vi "Pre Launch Init.vi"(11 "TableLogger_CSV_Actor in":refnum<class "TableLogger_CSV_Actor.lvclass">) -> (0 "error out":errorcluster, 3 "TableLogger_CSV_Actor out":refnum<class "TableLogger_CSV_Actor.lvclass">)   [LabVIEW 2014, in "TableLogger_CSV_Actor.lvlib" / "TableLogger_CSV_Actor.lvclass"]
doc: "(<B>Filename</B>: Actor Framework.lvlib:Actor.lvclass:Pre Launch Init.vi)\n\nDefines behavior that occurs after the Launch Nested Actor method is invoked but before the actor's Actor Core method begins running.\n\nBy default, this method does nothing. A descendant class may override it to define behavior."
uses:
  TableLogger_CSV_Actor.lvclass
  TableLogger_CSV_Actor.lvclass/TableLogger_CSV_Actor.ctl
  <userlib>/_OpenG.lib/file/file.llb/Strip Path - Traditional__ogtk.vi
  <userlib>/_OpenG.lib/file/file.llb/File Exists - Scalar__ogtk.vi
  <userlib>/_OpenG.lib/file/file.llb/Build Path - Traditional__ogtk.vi
  TableLogger_Actor/TableLogger_Actor/TableLogger_Actor.lvclass
panel:
  # "Connector Pane"
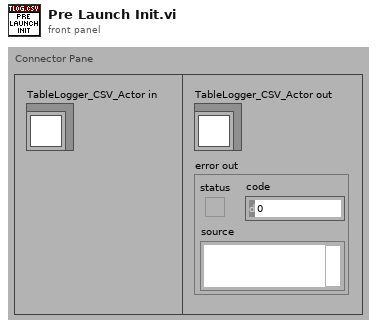
[diagram p1: front panel]
types:
  T1 = typedef "TableLogger_Actor.lvlib/TableLoggerConfig.ctl" = cluster{"TableLogger":T2, "DB File Path":path, "DB Backup Config":T3}
  T2 = typedef "TableLogger_Actor.lvlib/TableLoggerTypes.ctl" = enum16{"CSV Logger", "SQLite Logger"}
  T3 = typedef "TableLogger_Actor.lvlib/TableLoggerBackupConfig.ctl" = cluster{"Directory":path, "UTC Time Format":bool, "On Launch":bool, "Interval (Hours)":dbl, "Size Multiples (Bytes)":i32}
  T4 = typedef "Type Descriptor Enumeration__ogtk.ctl" = enum8{"<Null>", "I8", "I16", "I32", "I64", "U8", "U16", "U32", "U64", "SGL", "DBL", "EXT", "CSG", "CDB", "CXT", "0x0F", "0x10", "0x11", "0x12", "0x13", "0x14", "Enum U8", "Enum U16", "Enum U32", "Enum U64", "SGL PQ", "DBL PQ", "EXT PQ", "CSG PQ", "CDB PQ", "CXT PQ", "0x1F", "0x20", "Boolean", "0x22", "0x23", "0x24", "0x25", "0x26", "0x27", "0x28", "0x29", "0x2A", "0x2B", "0x2C", "0x2D", "0x2E", "0x2F", "String", "0x31", "Path", "Pict", "0x34", "0x35", "0x36", "DAQ", "0x38", "0x39", "0x3A", "0x3B", "0x3C", "0x3D", "0x3E", "0x3F", "Array", "0x41", "0x42", "0x43", "0x44", "0x45", "0x46", "0x47", "0x48", "0x49", "0x4A", "0x4B", "0x4C", "0x4D", "0x4E", "0x4F", "Cluster", "0x51", "0x52", "Variant", "Waveform", "0x55", "0x56", "0x57", "0x58", "0x59", "0x5A", "0x5B", "0x5C", "0x5D", "0x5E", "0x5F", "0x60", "0x61", "0x62", "0x63", "0x64", "0x65", "0x66", "0x67", "0x68", "0x69", "0x6A", "0x6B", "0x6C", "0x6D", "0x6E", "0x6F", "Refnum"}
  T5 = enum16{"open", "replace", "create", "open or create", "replace or create", "replace or create with confirmation"}
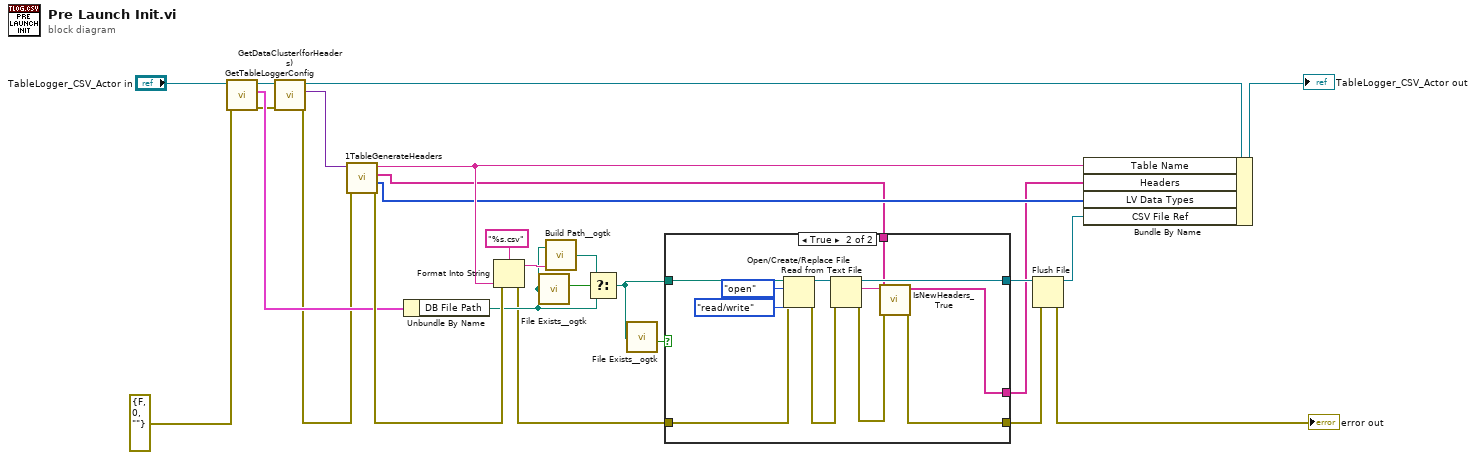
[diagram p0: block diagram]
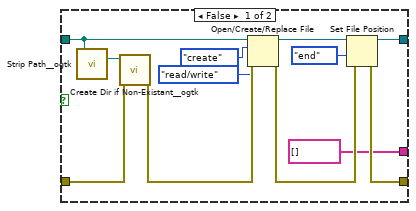
[diagram p2: hidden frame]
diagram:
  n1 = call-dynamic "GetTableLoggerConfig.vi"("error in (no error)"=errorcluster {"status"=FALSE, "code"=0, "source"=""}, "object in"="TableLogger_CSV_Actor in") -> ("error out"=w3:errorcluster, "TableLogger Config"=w5:T1, "object out"=w6:refnum<class "TableLogger_CSV_Actor.lvclass">)  [unwired: 7 in]
  n2 = call "GetDataCluster(forHeaders).vi"("error in (no error)"=w3, "object in"=w6) -> ("error out"=w1:errorcluster, "Data Cluster (for Headers)"=w4:variant, "object out"=w7:refnum<class "TableLogger_CSV_Actor.lvclass">)  [unwired: 7 in]
  n3 = call "1TableGenerateHeaders.vi"("error in (no error)"=w1, "Cluster Variant"=w4) -> ("error out"=w20:errorcluster, "LV Data Types"=w15:T4[], "Headers"=w12:string[], "Table Name"=w19:string)  [unwired: 6 in]
  n4 = Unbundle By Name(w5) -> ("DB File Path"=w18:path)
  n5 = Format Into String(format string="%s.csv", error in=w20, w19) -> (resulting string=w23:string, error out=w17:errorcluster)  [unwired: 1 in]
  n6 = call-poly <userlib>:"File Exists__ogtk.vi"("file path"=w18) -> ("is directory"=w24:bool)  [unwired: 6 in, 1 out]
  n7 = call-poly <userlib>:"Build Path__ogtk.vi"("name or relative path"=w23, "base path"=w18) -> ("appended path"=w21:path)
  n8 = Select(t=w21, s=w24, f=w18) -> (s? t:f=w14:path)
  n9 = call-poly <userlib>:"File Exists__ogtk.vi"("file path"=w14) -> ("exists"=w13:bool)  [unwired: 6 in, 1 out]
  n10 = case shown="True" w13 {
    tunnel: w17 -> [w36 w47]
    tunnel: [w28 w40] -> w11
    tunnel: [w30 w42] -> w10
    tunnel: w14 -> [w33 w50]
    tunnel: w12 -> [_ w41]
    tunnel: [string[] [] ("Headers") w39] -> w9
    frame False {
      n11 = call-poly <userlib>:"Strip Path__ogtk.vi"("path"=w33) -> ("stripped path"=w37:path)  [unwired: 1 out]
      n12 = call <userlib>:"Create Dir if Non-Existant__ogtk.vi"("error in (no error)"=w36, "Directory Path"=w37) -> ("error out"=w35:errorcluster)  [unwired: 7 in, 2 out]
      n13 = Open/Create/Replace File(file path (use dialog)=w33, error in=w35, operation (0:open)=T5."create", access (0:read/write)=enum16{"read/write", "read-only", "write-only"}."read/write") -> (refnum out=w31:refnum<file>, error out=w29:errorcluster)  [unwired: 2 in, 1 out]
      n14 = Set File Position(refnum=w31, from (0:start)=enum16{"start", "end", "current"}."end", error in=w29) -> (refnum out=w30:refnum<file>, error out=w28:errorcluster)  [unwired: 1 in]
    }
    frame True {
      n15 = Open/Create/Replace File(file path (use dialog)=w50, error in=w47, operation (0:open)=T5."open", access (0:read/write)=enum16{"read/write", "read-only", "write-only"}."read/write") -> (refnum out=w46:refnum<file>, error out=w43:errorcluster)  [unwired: 2 in, 1 out]
      n16 = Read from Text File(file (use dialog)=w46, error in=w43) -> (refnum out=w42:refnum<file>, text=w44:string, error out=w45:errorcluster)  [unwired: 2 in, 1 out]
      n17 = call "IsNewHeaders_True.vi"("error in"=w45, "Headers"=w41, "Data"=w44) -> ("error out"=w40:errorcluster, "Old Headers"=w39:string[])  [unwired: 6 in, 1 out]
    }
  }
  n18 = Flush File(refnum=w10, error in=w11) -> (refnum out=w16:refnum<file>, error out=→"error out":errorcluster)
  n19 = Bundle By Name(cluster=w7, "Table Name"=w19, "Headers"=w9, "LV Data Types"=w15, "CSV File Ref"=w16) -> (→"TableLogger_CSV_Actor out":refnum<class "TableLogger_CSV_Actor.lvclass">)
